vi "TimeCompare.vi"(1 "Time Variable":u32, 2 "Base Time":u32, 3 "Timer":u32) -> (0 "Time Outcome":enum16{"In Time", "Out Time"}(ring))   [LabVIEW 2010]
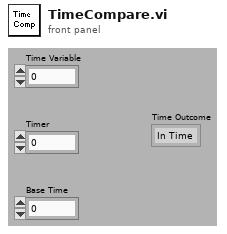
[diagram p1: front panel]
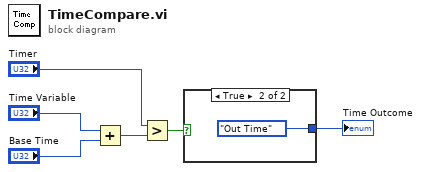
[diagram p0: block diagram]
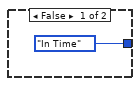
[diagram p2: hidden frame]
diagram:
  n1 = Add(x="Time Variable", y="Base Time") -> (x+y=w5:u32)
  n2 = Greater?(x="Timer", y=w5) -> (0:w3:bool)
  n3 = case shown="True" w3 {
    tunnel: [enum16{"In Time", "Out Time"}."In Time" ("Time Outcome") enum16{"In Time", "Out Time"}."Out Time" ("Time Outcome")] -> w1
    frame False {
    }
    frame True {
    }
  }
  "Time Outcome" <- w1
